vi "Chemyx_Syringe_Pump_AdvancedExample.vi"() -> ()   [LabVIEW 2016]
doc: "The advanced example uses a State Machine design pattern to demonstrate the upload and control of multiple steps of a Chemyx syringe pump."
uses:
  _driver/Basic driver/Status/controls/Pump_status_enum.ctl
  _driver/Basic driver/Communication/controls/comm_rate_enum.ctl
  controls/step_parameters.ctl
  _driver/Advanced driver/controls/unit_enum.ctl
  _driver/_private/Control/Control Mode.ctl
  _driver/_private/Control/Programmable Mode.ctl
  controls/advanced_example_states_enum.ctl
  <vilib>/Utility/miscctls.llb/LVStringsAndValuesArrayTypeDef_U16.ctl
  <vilib>/ErrorRing/Error Ring.xnode
  _driver/Chemyx_Syringe_Pump_driver.lvlib
panel:
  in  "Mode":T1=enum."Basic"
  in  "[x]":T2
  in  "Send settings":bool
  out "rate units":string="ml/min"
  out "Volume units":string="ml"
  in  "Diameter":dbl=12.5
  in  "Units":T3
  in  "Apply parameters":bool
  in  "Step parameters":T4={"Volume"=3.0, "time - min"=0, "time - sec"=0, "Rate"=1.0, "delay - min"=1, "delay - sec"=30} {"delay - sec" min=0 max=59; "delay - min" min=0 max=98; "Rate" min=0.0; "time - sec" min=0 max=59; "time - min" min=0 max=98}
  in  "Add step after":bool
  in  "Remove step":bool
  in  "Add step before":bool
  in  "Current step":u16(ring) items=["Step 1"]
  out "Connection":bool
  out "Limits":dbl[](array[numeric])
  in  "Baud rate":T5
  out "Status":T6
  in  "Quit Button":bool
  in  "Port":refnum<visa-resource-name>
  out "Dispensed volume":dbl
  out "Elapsed time":string
  in  "Reset Button":bool
  in  "Pause Button":bool
  in  "Stop Button":bool
  in  "Start Button":bool
  # "Multi-Steps"
  # "Communication Settings"
  # "Commands"
  # "Pump Status"
  # "mm"
  # "sec"
  # "Select Port and Baud rate before running the VI.\n\nThe advanced example uses a State Machine design pattern to demonstrate the upload and control of multiple steps of a Chemyx syringe pump."
  # "sec"
  # "Delay"
  # "min"
  # "Time"
  # "min"
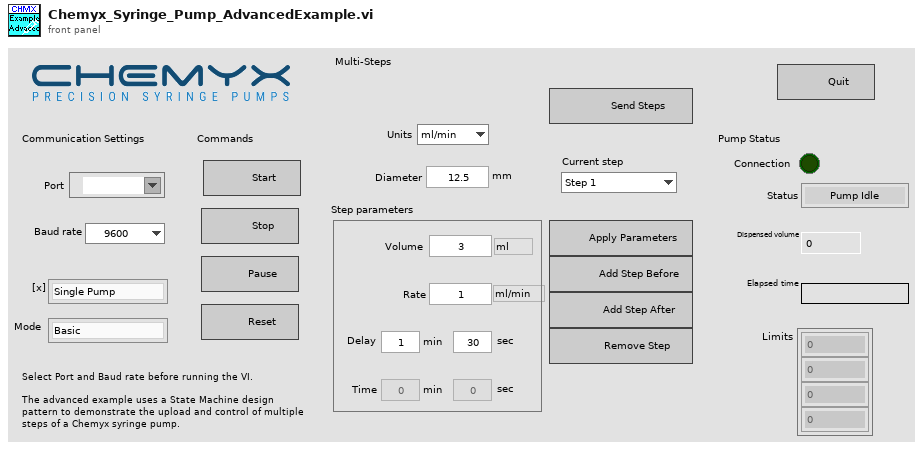
[diagram p1: front panel]
types:
  T1 = typedef "Chemyx_Syringe_Pump_driver.lvlib/Programmable Mode.ctl" = enum16{"Blank", "Basic", "Programmable"}
  T2 = typedef "Chemyx_Syringe_Pump_driver.lvlib/Control Mode.ctl" = enum16{"Single Pump", "Pump Channel 1", "Pump Channel 2", "Cycle Mode"}
  T3 = typedef "Chemyx_Syringe_Pump_driver.lvlib/unit_enum.ctl" = enum16{"ml/min", "ml/hr", "ul/min", "ul/hr"}
  T4 = typedef "step_parameters.ctl" = cluster{"Volume":dbl, "time - min":i32, "time - sec":i32, "Rate":dbl, "delay - min":i32, "delay - sec":i32}
  T5 = typedef "Chemyx_Syringe_Pump_driver.lvlib/comm_rate_enum.ctl" = enum16{"9600", "38400"}
  T6 = typedef "Chemyx_Syringe_Pump_driver.lvlib/Pump_status_enum.ctl" = enum16{"Pump Idle", "Pump Running", "Pump Paused", "Pump Delay", "Pump Stalled", "Pump Error"}
  T7 = cluster{"Connection":bool, "Step param array":T4[], "Status":T6, "Current UI step":u16, "Step parameter":T4, "Comm port":refnum<visa-resource-name>, "Units":T3, "Diameter":dbl, "Delay":dbl, "[x]":T2, "Mode":T1}
  T8 = typedef "advanced_example_states_enum.ctl" = enum16{"Initialize", "Wait for event", "Start", "Stop", "Pause", "Reset", "Add Step before", "Add Step After", "Remove Step", "Quit", "Error handling", "Change current step", "Send settings"}
  T9 = typedef "LVStringsAndValuesArrayTypeDef_U16.ctl" = cluster{"String":string, "Value":u16}[]
  T10 = enum16{"Left Button", "Center Button", "Right Button", "Window Close"}
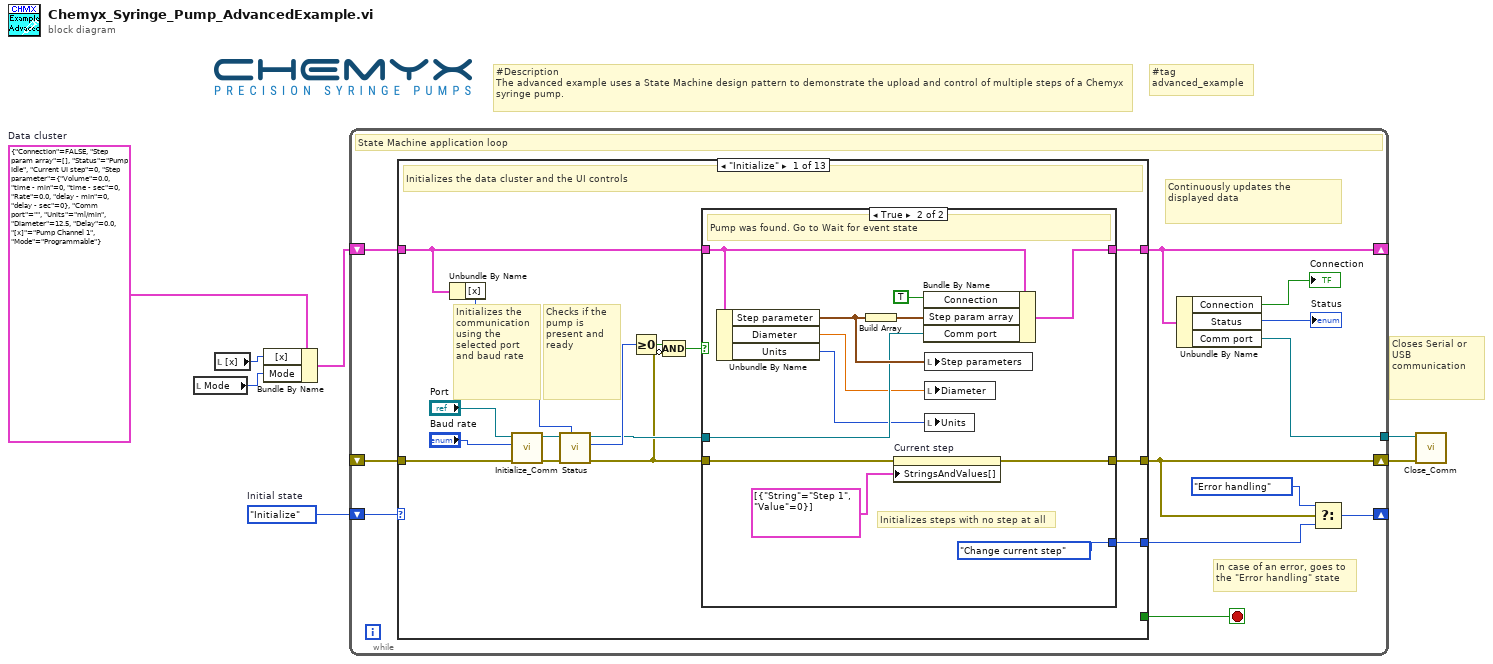
[diagram p0: block diagram]
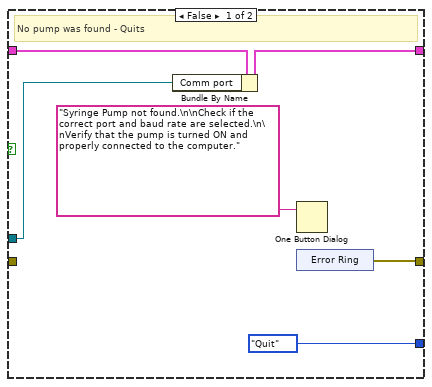
[diagram p2: hidden frame]
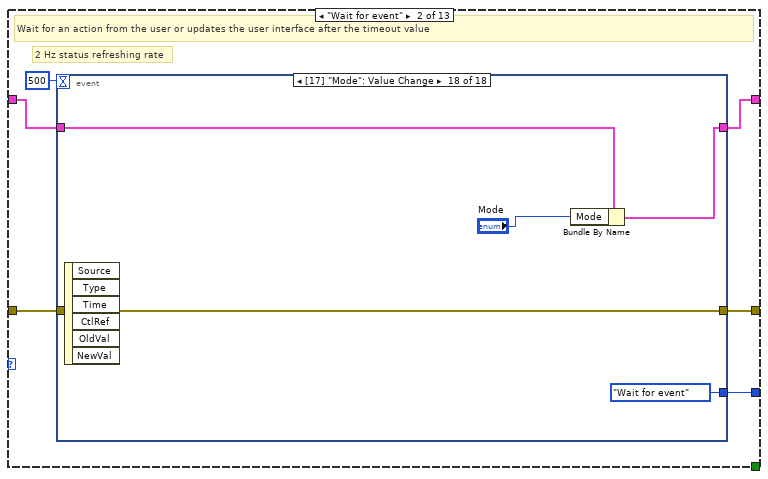
[diagram p3: hidden frame]
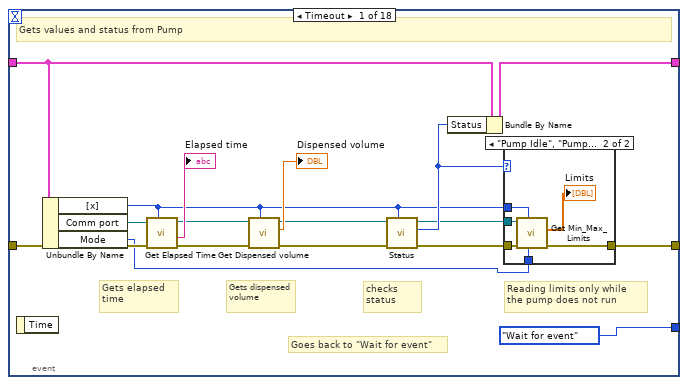
[diagram p4: hidden frame]
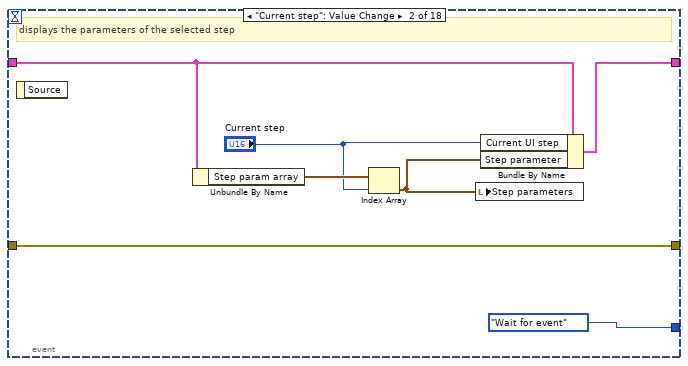
[diagram p6: hidden frame]
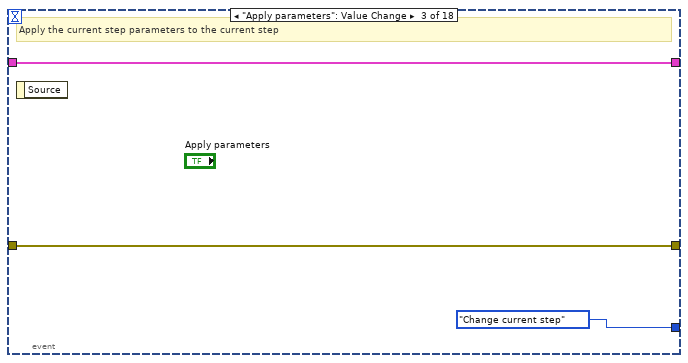
[diagram p7: hidden frame]
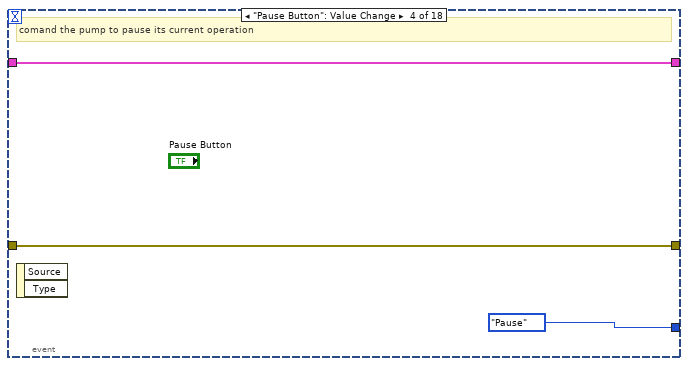
[diagram p8: hidden frame]
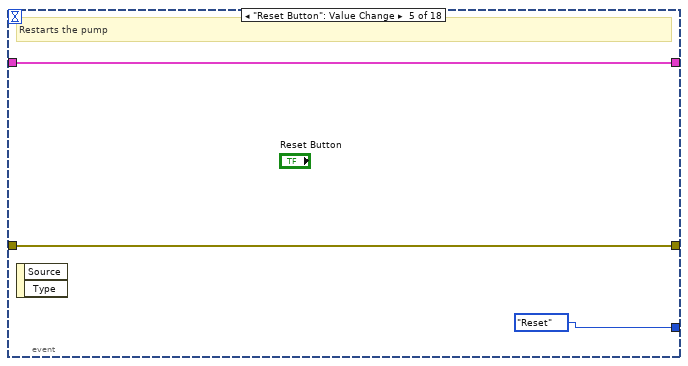
[diagram p9: hidden frame]
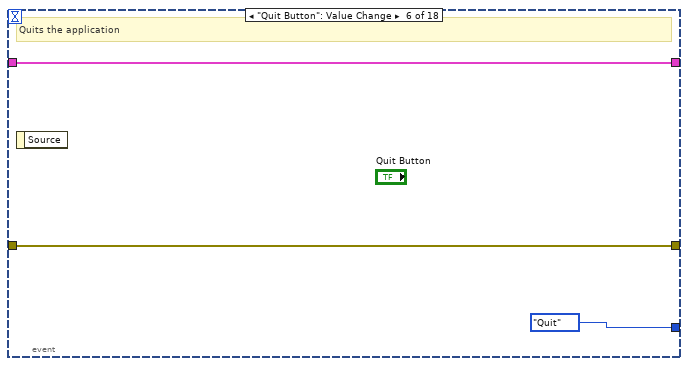
[diagram p10: hidden frame]
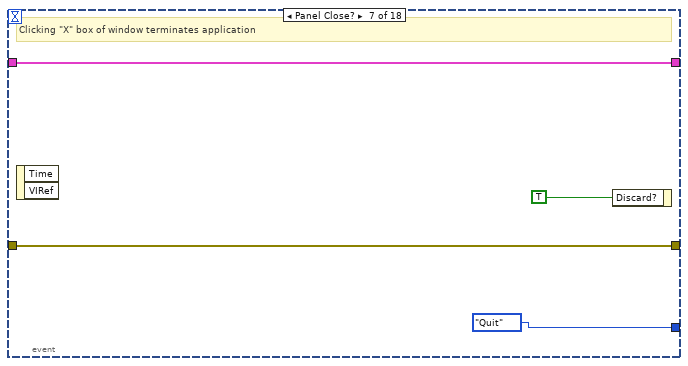
[diagram p11: hidden frame]
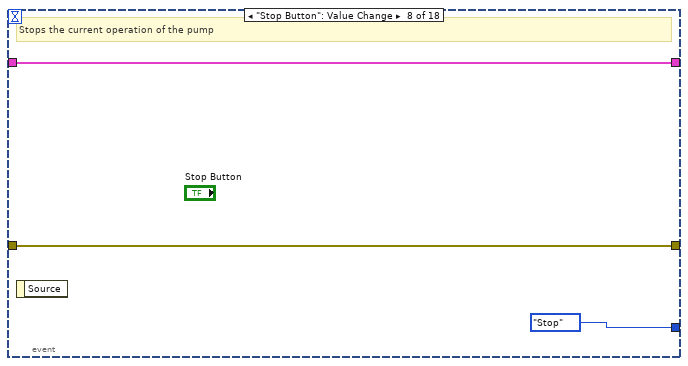
[diagram p12: hidden frame]
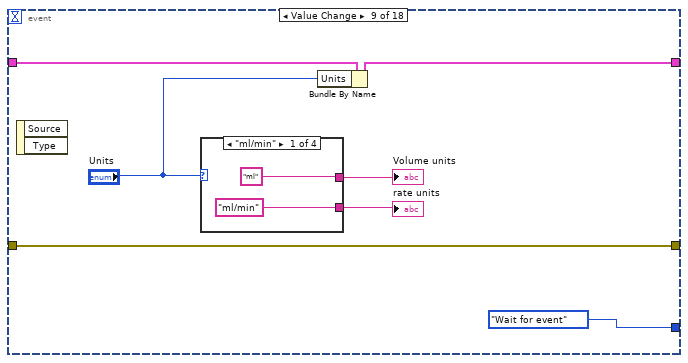
[diagram p13: hidden frame]
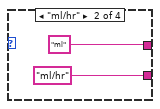
[diagram p14: hidden frame]
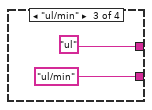
[diagram p15: hidden frame]
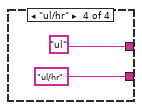
[diagram p16: hidden frame]
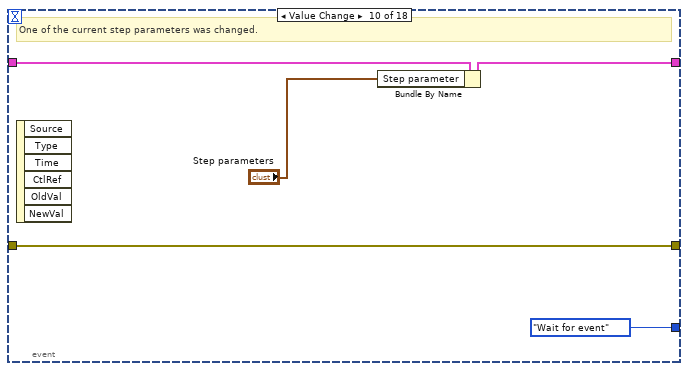
[diagram p17: hidden frame]
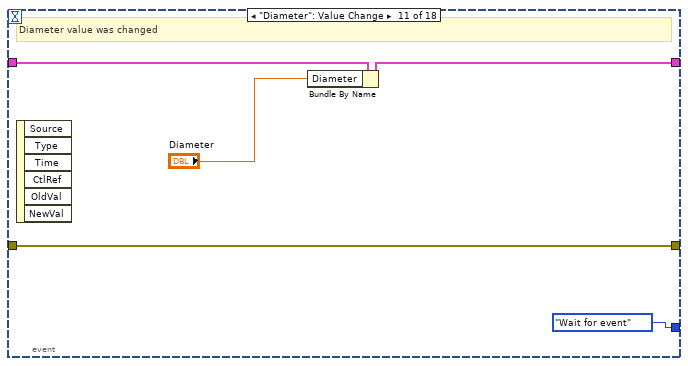
[diagram p18: hidden frame]
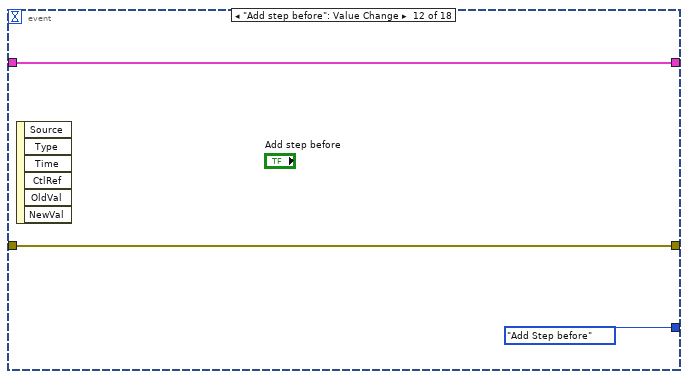
[diagram p19: hidden frame]
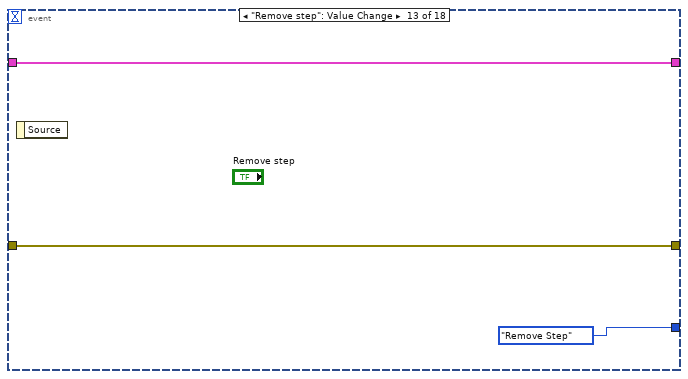
[diagram p20: hidden frame]
diagram:
  w4 = T7 {"Connection"=FALSE, "Step param array"=[], "Status"=enum."Pump Idle", "Current UI step"=0, "Step parameter"={"Volume"=0.0, "time - min"=0, "time - sec"=0, "Rate"=0.0, "delay - min"=0, "delay - sec"=0}, "Comm port"="", "Units"=enum."ml/min", "Diameter"=12.5, "Delay"=0.0, "[x]"=enum."Pump Channel 1", "Mode"=enum."Programmable"}  # Data cluster
  w6 = advanced_example_states_enum."Initialize"  # Initial state
  # "#tag\nadvanced_example"
  # "#Description\nThe advanced example uses a State Machine design pattern to demonstrate the upload and control of multiple steps of a Chemyx syringe pump."
  # "Closes Serial or USB communication"
  n1 = local read "Mode"() -> (w2:T1)
  n2 = local read "[x]"() -> (w3:T2)
  n3 = Bundle By Name(cluster=w4, "[x]"=w3, "Mode"=w2) -> (w1:T7)
  n4 = while {
    shift-right: [w13] -> w7
    shift-left: _ -> [w19]
    shift-right: [w10] -> _
    shift-left: w6 -> [w18]
    shift-right: [w15] -> _
    shift-left: w1 -> [w16]
    tunnel: [w8] -> w5
    stop <- w17 stop-if-true
    # "In case of an error, goes to the \"Error handling\" state"
    # "Continuously updates the displayed data"
    # "State Machine application loop"
    n5 = case shown="\"Initialize\"" w18 {
      tunnel: w19 -> [w28 w59 w164 w186 w200 w206 w211 w219 w231 w246 w265 w295 w307]
      tunnel: [w26 w57 w165 w168 w198 w204 w212 w217 w234 w244 w264 w294 w303] -> w13
      tunnel: [_ _ _ _ _ _ _ _ _ _ _ TRUE _] -> w17
      tunnel: [w23 w56 advanced_example_states_enum."Wait for event" advanced_example_states_enum."Wait for event" advanced_example_states_enum."Wait for event" advanced_example_states_enum."Wait for event" advanced_example_states_enum."Wait for event" advanced_example_states_enum."Wait for event" advanced_example_states_enum."Wait for event" advanced_example_states_enum."Wait for event" advanced_example_states_enum."Wait for event" advanced_example_states_enum."Quit" w304] -> w12
      tunnel: w16 -> [w21 w55 w163 w184 w199 w205 w210 w229 w238 w256 w259 w297 w308]
      tunnel: [w22 w54 w163 w184 w199 w205 w210 w216 w233 w243 w263 w292 w308] -> w15
      frame "Initialize" {
        # "Checks if the pump is present and ready"
        # "Initializes the communication using the selected port and baud rate"
        # "Initializes the data cluster and the UI controls"
        n6 = Unbundle By Name(w21) -> ("[x]"=w20:T2)
        n7 = call "Initialize_Comm.vi"("error in (no error)"=w28, "Baud rate"="Baud rate", "Serial Port in"="Port") -> ("error out"=w31:errorcluster, "Serial Port out"=w32:refnum<visa-resource-name>)  [unwired: 7 in]
        n8 = call "Status.vi"("[x]"=w20, "error in (no error)"=w31, "Serial Port in"=w32) -> ("error out"=w25:errorcluster, "Status"=w33:T6, "Serial Port out"=w27:refnum<visa-resource-name>)  [unwired: 6 in]
        n9 = Greater Or Equal To 0?(x=w33) -> (x >= 0?=w34:bool)
        n10 = Compound Arithmetic op=AND(w34, invert w25) -> (w29:bool)
        n11 = case shown="True" w29 {
          tunnel: w27 -> [w36 w44]
          tunnel: [w35 w50] -> w26
          tunnel: w25 -> [_ w51]
          tunnel: [advanced_example_states_enum."Quit" advanced_example_states_enum."Change current step"] -> w23
          tunnel: w21 -> [w38 w47]
          tunnel: [w37 w49] -> w22
          frame False {
            # "No pump was found - Quits"
            n12 = Bundle By Name(cluster=w38, "Comm port"=w36) -> (w37:T7)
            n13 = One Button Dialog(message="Syringe Pump not found.\n\nCheck if the correct port and baud rate are selected.\n\nVerify that the pump is turned ON and properly connected to the computer.") -> ()  [unwired: 1 in, 1 out]
            n14 = xnode "Error Ring"() -> ("error out"=w35:errorcluster)
          }
          frame True {
            # "Initializes steps with no step at all"
            # "Pump was found. Go to Wait for event state"
            n15 = Unbundle By Name(w47) -> ("Step parameter"=w45:T4, "Diameter"=w42:dbl, "Units"=w43:T3)
            n16 = Build Array(w45) -> (w46:T4[])
            n17 = property on="Current step" class="Ring (strict)"(error in=w51, "StringsAndValues[]"=T9 [{"String"="Step 1", "Value"=0}] ("Strings And Values []")) -> (error out=w50:errorcluster)  [unwired: 1 in, 1 out]
            n18 = Bundle By Name(cluster=w47, "Connection"=TRUE, "Step param array"=w46, "Comm port"=w44) -> (w49:T7)
            n19 = local write "Step parameters"(w45) -> ()
            n20 = local write "Diameter"(w42) -> ()
            n21 = local write "Units"(w43) -> ()
          }
        }
      }
      frame "Wait for event" {
        # "2 Hz status refreshing rate"
        # "Wait for an action from the user or updates the user interface after the timeout value"
        n22 = event shown="[17] \"Mode\": Value Change" {
          selector: _ -> [_ _ _ _ _ _ _ _ _ _ _ _ _ _ _ _ _ _]
          dyn-events: _ -> [_ _ _ _ _ _ _ _ _ _ _ _ _ _ _ _ _ _]
          timeout: 500 -> [_ _ _ _ _ _ _ _ _ _ _ _ _ _ _ _ _ _]
          tunnel: w59 -> [w63 w88 w93 w94 w97 w102 w105 w109 w116 w129 w134 w137 w140 w143 w146 w149 w154 w159]
          tunnel: [w72 w88 w93 w94 w97 w102 w105 w109 w116 w129 w134 w137 w140 w143 w146 w149 w154 w159] -> w57
          tunnel: [advanced_example_states_enum."Wait for event" advanced_example_states_enum."Wait for event" advanced_example_states_enum."Change current step" advanced_example_states_enum."Pause" advanced_example_states_enum."Reset" advanced_example_states_enum."Quit" advanced_example_states_enum."Quit" advanced_example_states_enum."Stop" advanced_example_states_enum."Wait for event" advanced_example_states_enum."Wait for event" advanced_example_states_enum."Wait for event" advanced_example_states_enum."Add Step before" advanced_example_states_enum."Remove Step" advanced_example_states_enum."Add Step After" advanced_example_states_enum."Start" advanced_example_states_enum."Send settings" advanced_example_states_enum."Wait for event" advanced_example_states_enum."Wait for event"] -> w56
          tunnel: w55 -> [w69 w90 w92 w95 w99 w100 w103 w107 w112 w128 w133 w136 w139 w142 w145 w148 w153 w158]
          tunnel: [w70 w86 w92 w95 w99 w100 w103 w107 w111 w127 w132 w136 w139 w142 w145 w148 w151 w157] -> w54
          event Timeout {
            # "Goes back to \"Wait for event\""
            # "Gets dispensed volume"
            # "Gets elapsed time"
            # "checks status"
            # "Reading limits only while the pump does not run"
            # "Gets values and status from Pump"
            n23 = event-data() -> ()  [unwired: 1 in, 1 out]
            n24 = Unbundle By Name(w69) -> ("[x]"=w61:T2, "Comm port"=w64:refnum<visa-resource-name>, "Mode"=w60:T1)
            n25 = call "Get Elapsed Time.vi"("[x]"=w61, "error in (no error)"=w63, "Serial Port in"=w64) -> ("error out"=w76:errorcluster, "Time string"=→"Elapsed time":string, "Serial Port out"=w74:refnum<visa-resource-name>)  [unwired: 6 in]
            n26 = call "Get Dispensed volume.vi"("[x]"=w61, "error in (no error)"=w76, "Serial Port in"=w74) -> ("error out"=w67:errorcluster, "Volume"=→"Dispensed volume":dbl, "Serial Port out"=w62:refnum<visa-resource-name>)  [unwired: 6 in]
            n27 = call "Status.vi"("[x]"=w61, "error in (no error)"=w67, "Serial Port in"=w62) -> ("error out"=w66:errorcluster, "Status"=w68:T6, "Serial Port out"=w65:refnum<visa-resource-name>)  [unwired: 6 in]
            n28 = Bundle By Name(cluster=w69, "Status"=w68) -> (w70:T7)
            n29 = case shown="\"Pump Idle\", \"Pump Paused\", \"Pump Delay\"" w68 {
              tunnel: w66 -> [w77 w83]
              tunnel: [w77 w82] -> w72
              tunnel: w65 -> [_ w81]
              tunnel: w61 -> [_ w79]
              tunnel: w60 -> [_ w78]
              frame "Pump Running", Default {
              }
              frame "Pump Idle", "Pump Paused", "Pump Delay" {
                n30 = call "Get Min_Max_Limits.vi"("Mode"=w78, "[x]"=w79, "error in (no error)"=w83, "Serial Port in"=w81) -> ("error out"=w82:errorcluster, "Limits"=→"Limits":dbl[])  [unwired: 5 in, 1 out]
              }
            }
          }
          event "Current step": Value Change {
            # "displays the parameters of the selected step"
            n31 = event-data() -> ()  [unwired: 1 in, 1 out]
            n32 = Unbundle By Name(w90) -> ("Step param array"=w89:T4[])
            n33 = Index Array(array=w89, index="Current step") -> (element=w84:T4)
            n34 = local write "Step parameters"(w84) -> ()
            n35 = Bundle By Name(cluster=w90, "Current UI step"="Current step", "Step parameter"=w84) -> (w86:T7)
          }
          event "Apply parameters": Value Change {
            # "Apply the current step parameters to the current step"
            n36 = event-data() -> ()  [unwired: 1 in, 1 out]
          }
          event "Pause Button": Value Change {
            # "comand the pump to pause its current operation"
            n37 = event-data() -> ()  [unwired: 1 in, 2 out]
          }
          event "Reset Button": Value Change {
            # "Restarts the pump"
            n38 = event-data() -> ()  [unwired: 1 in, 2 out]
          }
          event "Quit Button": Value Change {
            # "Quits the application"
            n39 = event-data() -> ()  [unwired: 1 in, 1 out]
          }
          event Panel Close? {
            # "Clicking \"X\" box of window terminates application"
            n40 = event-data() -> ()  [unwired: 1 in, 2 out]
            n41 = event-data("Discard?"=TRUE) -> ()  [unwired: 1 in, 1 out]
          }
          event "Stop Button": Value Change {
            # "Stops the current operation of the pump"
            n42 = event-data() -> ()  [unwired: 1 in, 1 out]
          }
          event Value Change {
            n43 = event-data() -> ()  [unwired: 1 in, 2 out]
            n44 = case shown="\"ml/min\"" "Units" {
              tunnel: ["ml" ("Volume units") "ml" ("Volume units") "ul" ("Volume units") "ul" ("Volume units")] -> w113
              tunnel: ["ml/min" ("Volume units") "ml/hr" ("Volume units") "ul/min" ("Volume units") "ul/hr" ("Volume units")] -> w114
              frame "ml/min" {
              }
              frame "ml/hr" {
              }
              frame "ul/min" {
              }
              frame "ul/hr" {
              }
            }
            "Volume units" <- w113
            "rate units" <- w114
            n45 = Bundle By Name(cluster=w112, "Units"="Units") -> (w111:T7)
          }
          event Value Change {
            # "One of the current step parameters was changed."
            n46 = event-data() -> ()  [unwired: 1 in, 6 out]
            n47 = Bundle By Name(cluster=w128, "Step parameter"="Step parameters") -> (w127:T7)
          }
          event "Diameter": Value Change {
            # "Diameter value was changed"
            n48 = event-data() -> ()  [unwired: 1 in, 6 out]
            n49 = Bundle By Name(cluster=w133, "Diameter"="Diameter") -> (w132:T7)
          }
          event "Add step before": Value Change {
            n50 = event-data() -> ()  [unwired: 1 in, 6 out]
          }
          event "Remove step": Value Change {
            n51 = event-data() -> ()  [unwired: 1 in, 1 out]
          }
          event "Add step after": Value Change {
            n52 = event-data() -> ()  [unwired: 1 in, 2 out]
          }
          event "Start Button": Value Change {
            # "Starts the currently selected operation of the pump"
            n53 = event-data() -> ()  [unwired: 1 in, 1 out]
          }
          event "Send settings": Value Change {
            # "Go to send setting case"
            # "Received command to send the settings to the pump."
            n54 = event-data() -> ()  [unwired: 1 in, 6 out]
          }
          event Value Change {
            n55 = event-data() -> ()  [unwired: 1 in, 6 out]
            n56 = Bundle By Name(cluster=w153, "[x]"="[x]") -> (w151:T7)
          }
          event Value Change {
            n57 = event-data() -> ()  [unwired: 1 in, 6 out]
            n58 = Bundle By Name(cluster=w158, "Mode"="Mode") -> (w157:T7)
          }
        }
      }
      frame "Start" {
        # "Starts the pump"
        # "Starts the pumping operations using the current settings of the pump"
        n59 = Unbundle By Name(w163) -> ("[x]"=w161:T2, "Comm port"=w162:refnum<visa-resource-name>, "Mode"=w160:T1)
        n60 = call "Start.vi"("Mode"=w160, "[x]"=w161, "error in (no error)"=w164, "Serial Port in"=w162) -> ("error out"=w165:errorcluster)  [unwired: 6 in, 1 out]
      }
      frame "Send settings" {
        # "Sets rates for each step"
        # "Sets volumes for each step"
        # "Sets the delay before actual operation"
        # "Sets the syringe diameter"
        # "applies the selected units"
        # "Sends the parameters of all the steps."
        # "converts to minutes"
        # "Sends the settings and parameters of all steps to the pump."
        n61 = Unbundle By Name(w184) -> ("Step param array"=w181:T4[], "Diameter"=w182:dbl, "Comm port"=w180:refnum<visa-resource-name>, "Units"=w183:T3, "[x]"=w167:T2)  [unwired: 1 out]
        n62 = call "Set units.vi"("[x]"=w167, "error in (no error)"=w186, "Units"=w183, "Serial Port in"=w180) -> ("error out"=w178:errorcluster, "Serial Port out"=w179:refnum<visa-resource-name>)  [unwired: 6 in]
        n63 = for {
          tunnel: w181 -> [w196] mode=indexing
          tunnel: [w195] -> w177 mode=indexing
          tunnel: [w194] -> w175 mode=indexing
          tunnel: [w193] -> w172 mode=indexing
          n64 = Unbundle By Name(w196) -> ("delay - min"=w189:i32, "delay - sec"=w191:i32, "Rate"=w194:dbl, "Volume"=w195:dbl)
          n65 = To Double Precision Float(number=w189) -> (double precision float=w188:dbl)
          n66 = To Double Precision Float(number=w191) -> (double precision float=w187:dbl)
          n67 = Divide(x=w187, y=60.0) -> (x/y=w192:dbl)
          n68 = Add(x=w188, y=w192) -> (x+y=w193:dbl)
        }
        n69 = call "Set diameter.vi"("[x]"=w167, "error in (no error)"=w178, "Diameter (mm)"=w182, "Serial Port in"=w179) -> ("error out"=w170:errorcluster, "Serial Port out"=w169:refnum<visa-resource-name>)  [unwired: 6 in]
        n70 = call "Set volume.vi"("[x]"=w167, "error in (no error)"=w170, "Volume (array)"=w177, "Serial Port in"=w169) -> ("error out"=w176:errorcluster, "Serial Port out"=w174:refnum<visa-resource-name>)  [unwired: 6 in]
        n71 = call "Set rate.vi"("[x]"=w167, "error in (no error)"=w176, "Rate (array)"=w175, "Serial Port in"=w174) -> ("error out"=w171:errorcluster, "Serial Port out"=w173:refnum<visa-resource-name>)  [unwired: 6 in]
        n72 = call "Set delay.vi"("[x]"=w167, "error in (no error)"=w171, "Delay (min)"=w172, "Serial Port in"=w173) -> ("error out"=w168:errorcluster)  [unwired: 6 in, 1 out]
      }
      frame "Stop" {
        # "Stops the VI."
        n73 = Unbundle By Name(w199) -> ("[x]"=w197:T2, "Comm port"=w201:refnum<visa-resource-name>)
        n74 = call "Stop.vi"("[x]"=w197, "error in (no error)"=w200, "Serial Port in"=w201) -> ("error out"=w198:errorcluster)  [unwired: 7 in, 1 out]
      }
      frame "Pause" {
        # "Pauses the current Pump operation."
        n75 = Unbundle By Name(w205) -> ("[x]"=w203:T2, "Comm port"=w207:refnum<visa-resource-name>)
        n76 = call "Pause.vi"("[x]"=w203, "error in (no error)"=w206, "Serial Port in"=w207) -> ("error out"=w204:errorcluster)  [unwired: 7 in, 1 out]
      }
      frame "Reset" {
        # "Restarts the pump."
        n77 = Unbundle By Name(w210) -> ("Comm port"=w209:refnum<visa-resource-name>)
        n78 = call "Reset.vi"("error in (no error)"=w211, "Serial Port in"=w209) -> ("error out"=w212:errorcluster)  [unwired: 8 in, 1 out]
      }
      frame "Add Step before" {
        # "Add a step before the currently selected step."
        n79 = Unbundle By Name(w229) -> ("Step param array"=w228:T4[], "Current UI step"=w218:u16, "Step parameter"=w227:T4)
        n80 = property on="Current step" class="Ring (strict)"(error in=w219) -> (error out=w220:errorcluster, "Strings []"=w226:string[])  [unwired: 1 in, 1 out]
        n81 = Array Size(array=w226) -> (size(s)=w224:i32)
        n82 = Increment(x=w224) -> (x+1=w214:i32)
        n83 = Number To Decimal String(number=w214) -> (decimal integer string=w223:string)  [unwired: 1 in]
        n84 = Concatenate Strings("Step " ("string"), w223) -> (w222:string)
        n85 = Build Array (concatenate)(w226, w222) -> (w221:string[])
        n86 = property on="Current step" class="Ring (strict)"(error in=w220, "Strings []"=w221, "Value"=w218) -> (error out=w217:errorcluster)  [unwired: 1 in, 1 out]
        n87 = Insert Into Array(array=w228, index=w218, new element=w227) -> (w215:T4[])
        n88 = Bundle By Name(cluster=w229, "Step param array"=w215) -> (w216:T7)
      }
      frame "Change current step" {
        # "display the parameters of the newly selected step"
        n89 = Unbundle By Name(w238) -> ("Step param array"=w237:T4[], "Current UI step"=w235:u16, "Step parameter"=w236:T4)
        n90 = Replace Array Subset(array=w237, new element=w236, index=w235) -> (w232:T4[])
        n91 = property on="Current step" class="Ring (strict)"(error in=w231, "Value"=w235) -> (error out=w234:errorcluster)  [unwired: 1 in, 1 out]
        n92 = Bundle By Name(cluster=w238, "Step param array"=w232) -> (w233:T7)
      }
      frame "Add Step After" {
        # "adds a step after the currently selected step."
        n93 = property on="Current step" class="Ring (strict)"(error in=w246) -> (error out=w247:errorcluster, "Strings []"=w253:string[])  [unwired: 1 in, 1 out]
        n94 = Unbundle By Name(w256) -> ("Step param array"=w255:T4[], "Current UI step"=w245:u16, "Step parameter"=w254:T4)
        n95 = Array Size(array=w253) -> (size(s)=w251:i32)
        n96 = Increment(x=w251) -> (x+1=w240:i32)
        n97 = Number To Decimal String(number=w240) -> (decimal integer string=w250:string)  [unwired: 1 in]
        n98 = Increment(x=w245) -> (x+1=w241:u16)
        n99 = Concatenate Strings("Step " ("string"), w250) -> (w249:string)
        n100 = Build Array (concatenate)(w253, w249) -> (w248:string[])
        n101 = property on="Current step" class="Ring (strict)"(error in=w247, "Strings []"=w248, "Value"=w241) -> (error out=w244:errorcluster)  [unwired: 1 in, 1 out]
        n102 = Insert Into Array(array=w255, index=w241, new element=w254) -> (w242:T4[])
        n103 = Bundle By Name(cluster=w256, "Step param array"=w242, "Current UI step"=w241) -> (w243:T7)
      }
      frame "Remove Step" {
        # "Removes the currently selected step unless it is the last one."
        n104 = Unbundle By Name(w259) -> ("Step param array"=w258:T4[])
        n105 = Array Size(array=w258) -> (size(s)=w261:i32)
        n106 = Greater?(x=w261, y=1) -> (0:w262:bool)
        n107 = case shown="True" w262 {
          tunnel: w259 -> [w269 w288]
          tunnel: w265 -> [w268 w283]
          tunnel: [w268 w282] -> w264
          tunnel: [w269 w281] -> w263
          frame False {
            n108 = One Button Dialog(message="Cannot remove step when only 1 step remains.") -> ()  [unwired: 1 in, 1 out]
          }
          frame True {
            # "Converted to signed integer so that the test <0 works"
            # "If 1st step is removed, the new 1st step is displayed."
            # "uses a Val(Sgnl) so that parameters get updated as well using the event structure."
            n109 = Unbundle By Name(w288) -> ("Step param array"=w287:T4[], "Current UI step"=w270:u16)
            n110 = property on="Current step" class="Ring (strict)"(error in=w283) -> (error out=w284:errorcluster, "Strings []"=w286:string[])  [unwired: 1 in, 1 out]
            n111 = Array Size(array=w286) -> (size(s)=w278:i32)
            n112 = To Word Integer(number=w270) -> (16bit integer=w271:i16)
            n113 = Decrement(x=w278) -> (x-1=w276:i32)
            n114 = Decrement(x=w271) -> (x-1=w272:i16)
            n115 = Array Subset(array=w286, index=0, length=w276) -> (w285:string[])
            n116 = Less Than 0?(x=w272) -> (x < 0?=w275:bool)
            n117 = Delete From Array(array=w287, length=1, index=w270) -> (array with subset deleted=w280:T4[])  [unwired: 1 out]
            n118 = Select(t=u16 0 ("x-1"), s=w275, f=w272) -> (s? t:f=w274:u16)
            n119 = Bundle By Name(cluster=w288, "Step param array"=w280, "Current UI step"=w274) -> (w281:T7)
            n120 = property on="Current step" class="Ring (strict)"(error in=w284, "Strings []"=w285, "Val(Sgnl)"=w274) -> (error out=w282:errorcluster)  [unwired: 1 in, 1 out]
          }
        }
      }
      frame "Quit" {
        # "Quits the application."
        n121 = Unbundle By Name(w297) -> ("[x]"=w289:T2, "Status"=w296:T6, "Comm port"=w290:refnum<visa-resource-name>)
        n122 = case shown="\"Pump Running\", \"Pump Paused\"" w296 {
          tunnel: w295 -> [w299 w302]
          tunnel: w290 -> [_ w301]
          tunnel: [w299 w300] -> w294
          tunnel: w289 -> [_ _]
          frame "Pump Idle", Default {
          }
          frame "Pump Running", "Pump Paused" {
            # "In case pump is still running,\nstops it before quitting the application"
            n123 = call "Stop.vi"("error in (no error)"=w302, "Serial Port in"=w301) -> ("error out"=w300:errorcluster)  [unwired: 8 in, 1 out]
          }
        }
        n124 = Bundle By Name(cluster=w297, "Connection"=FALSE) -> (w292:T7)
      }
      frame "Error handling" {
        # "Handles any error by providing a dialog to the user to continue, quit normally, or abort."
        n125 = Unbundle By Name(w307) -> ("code"=w306:i32, "source"=w305:string)
        n126 = case shown="1, Default" w306 {
          selector: w306 -> [_ w317]
          tunnel: w305 -> [_ w314]
          tunnel: [advanced_example_states_enum."Wait for event" w310] -> w304
          frame 85 {
            # "Error 85: data conversion error: Some command received from the pump are sometimes formatted wrong when the pump UI is used or the pump is running"
            # "Use this case to list the errors that you want to ignore"
          }
          frame 1, Default {
            # "Dialog also displays info about the error"
            # "Dialog for the user to choose to continue with the application, quit normally, or abort."
            n127 = Number To Decimal String(number=w317) -> (decimal integer string=w316:string)  [unwired: 1 in]
            n128 = Concatenate Strings("Error no. " ("Left Button Text (\"Yes\")"), w316, " Error details:\n" ("Left Button Text (\"Yes\")"), w314, "\n\nDo you want to Continue, Quit Normally, or Abort?" ("Left Button Text (\"Yes\")")) -> (w312:string)
            n129 = call <vilib>:"Three Button Dialog.vi"("Window Title (\"\")"="An error occurred" ("message"), "Right Button Text (\"Cancel\")"="Abort" ("Right Button Text (\"Cancel\")"), "Center Button Text (\"No\")"="Quit Normally" ("Center Button Text (\"No\")"), "Left Button Text (\"Yes\")"="Continue" ("Left Button Text (\"Yes\")"), "message"=w312) -> ("Which Button?"=w311:T10)  [unwired: 6 in]
            n130 = case shown="\"Right Button\"" w311 {
              tunnel: [advanced_example_states_enum."Wait for event" advanced_example_states_enum."Quit" advanced_example_states_enum."Error handling"] -> w310
              frame "Left Button", Default {
                # "Continue"
              }
              frame "Center Button" {
                # "Quit Normally"
              }
              frame "Right Button" {
                # "Abort"
                n131 = Stop() -> ()  [unwired: 1 in]
              }
            }
          }
        }
        n132 = xnode "Error Ring"() -> ("error out"=w303:errorcluster)
      }
    }
    n133 = Unbundle By Name(w15) -> ("Connection"=→"Connection":bool, "Status"=→"Status":T6, "Comm port"=w8:refnum<visa-resource-name>)
    n134 = Select(t=advanced_example_states_enum."Error handling", s=w13, f=w12) -> (s? t:f=w10:T8)
  }
  n135 = call "Close_Comm.vi"("error in (no error)"=w7, "Serial Port in"=w5) -> ()  [unwired: 9 in, 1 out]
